vi "helper-log-parse-irr.vi"(11 "output cluster":T1 {"clk" format="%#.3f"}) -> (2 "Cluster":cluster{"sample":dbl, "UV Limit":dbl}, 3 "update chart?":bool)   [LabVIEW 2024]
uses:
  controls/typeEngineLogCluster.ctl
  controls/type.StepFunction.ctl
  globals/globals-engine.vi
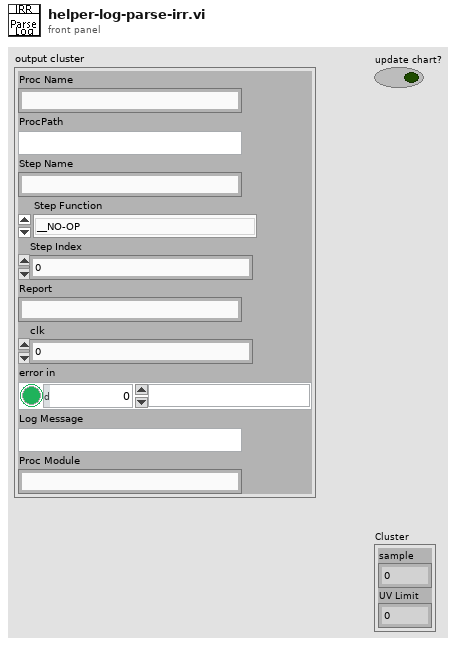
[diagram p1: front panel]
types:
  T1 = typedef "typeEngineLogCluster.ctl" = cluster{"Proc Name":string, "ProcPath":string, "Step Name":string, "Step Function":T2, "Step Index":i32, "Report":string, "clk":dbl, "error in":errorcluster, "Log Message":string, "Proc Module":string}
  T2 = typedef "type.StepFunction.ctl" = enum16{"__NO-OP", "_DELAY_LOAD", "_DELAY_COMPARE", "_JUMP", "_COMPLETE", "_COMPARE", "_LOG_MESSAGE", "_LOG_LAST_REPORT", "_SCHEDULE", "_SCHED_DAILY", "CLK_COMPARE", "PROC_START", "PROC_STOP", "PROC_LOAD", "PROC_COMPLETION_CHECK", "PROC_COMPLETION_LOAD", "_IO_READ", "_IO_READ_MANY", "_IO_WRITE", "_IO_WRITE_BY_REG", "_IO_GET_OUTPUT", "_OCS_CHECK", "_OCS_RECORD", "_GET_RH", "_GET_ACC_UV", "_GET_WD", "_GET_WS", "_REC_DELETE", "_REC_MOVE", "_REC_COPY", "_IRR_CHECK", "UNIT_CHECK", "UNIT_SAMPLE", "UNIT_DOSE"}
  T3 = typedef "irr-panel.ctl" = cluster{"Day Time":cluster{"Sunset":timestamp, "Sunrise":timestamp}, "timeLimits":cluster{"Irrigation":dbl, "Nut./Water":dbl}, "Calculated Timing":cluster{"Irrigation Timeout":timestamp, "Nutrients Timeout":timestamp}, "Irr Dosing Time":cluster{"Nutrients":u16, "Water":u16, "Wash":u16}, "UV Limit ":dbl, "Dose Table":cluster{"Enable":bool, "output":string}[], "Last Iteration":timestamp, "UV Reduction Status":bool, "UV Reduction":u8}
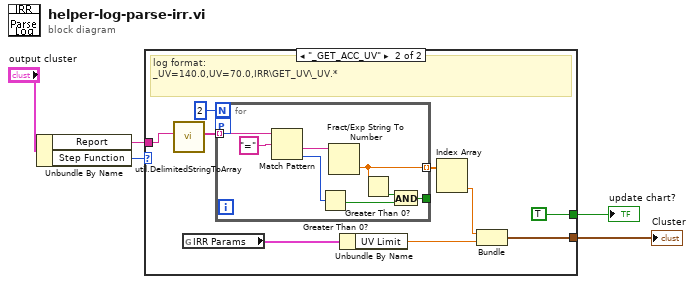
[diagram p0: block diagram]
diagram:
  n1 = Unbundle By Name("output cluster") -> ("Report"=w2:string, "Step Function"=w1:T2)
  n2 = case shown="\"_GET_ACC_UV\"" w1 {
    tunnel: w2 -> [_ w9]
    tunnel: [_ w7] -> w4
    tunnel: [_ TRUE] -> w5
    frame Default {
    }
    frame "_GET_ACC_UV" {
      # "log format: \n_UV=140.0,UV=70.0,IRR\\GET_UV\\_UV.*"
      n3 = call "util.DelimitedStringToArray.vi"("delimitaed string"=w9) -> ("array out"=w13:string[])  [unwired: 10 in]
      n4 = global read "globals-engine.vi" "IRR Params"() -> (w12:T3)
      n5 = for {
        N: 2 -> [_]
        tunnel: w13 -> [w21] mode=indexing
        tunnel: [w18] -> w14 mode=indexing
        tunnel: [w15] -> _
        workers-P: _ -> [_]
        n6 = Match Pattern(string=w21, regular expression="=") -> (after substring=w20:string, offset past match=w19:i32)  [unwired: 1 in, 2 out]
        n7 = Greater Than 0?(x=w19) -> (x > 0?=w16:bool)
        n8 = Fract/Exp String To Number(string=w20) -> (number=w18:dbl)  [unwired: 3 in, 1 out]
        n9 = Greater Than 0?(x=w18) -> (x > 0?=w17:bool)
        n10 = And(x=w17, y=w16) -> (x .and. y?=w15:bool)
      }
      n11 = Unbundle By Name(w12) -> ("UV Limit"=w11:dbl)
      n12 = Index Array(array=w14) -> (element #2=w8:dbl)  [unwired: 2 in, 1 out]
      n13 = Bundle(w8, "UV Limit"=w11) -> (w7:cluster{dbl, "UV Limit ":dbl})  [unwired: 1 in]
    }
  }
  "update chart?" <- w5
  "Cluster" <- w4
